vi "Polymorphic VI Experiment 1.vi"   [LabVIEW 2014]
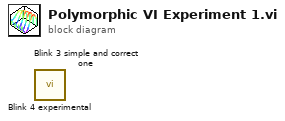
[diagram p0: block diagram]
diagram:
  n1 = call "Blink 4 experimental.vi"() -> ()  [unwired: 11 in, 1 out]
  n2 = call "Blink 3 simple and correct one.vi"() -> ()  [unwired: 10 in, 2 out]
